vi "chart add series lv.vi"(7 "y2_axis":u8, 8 "error in (no error)":errorcluster, 9 "values":string, 10 "categories":string, 11 "chart":u32) -> (0 "error out":errorcluster, 3 "function return":u32)   [LabVIEW 8.6]
doc: "lxw_chart_series chart_add_series_lv(lxw_chart chart, const char *categories, const char *values, uint8_t y2_axis);"
uses:
  pending_lvxlsxwriter/xlsxwriter.dll
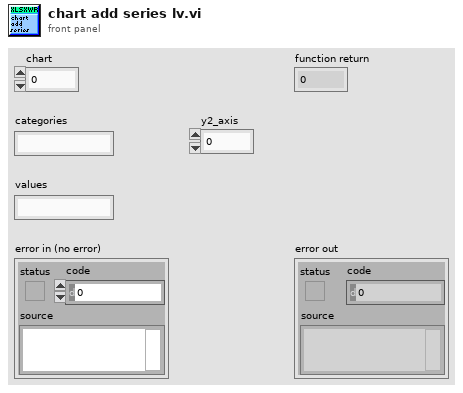
[diagram p1: front panel]
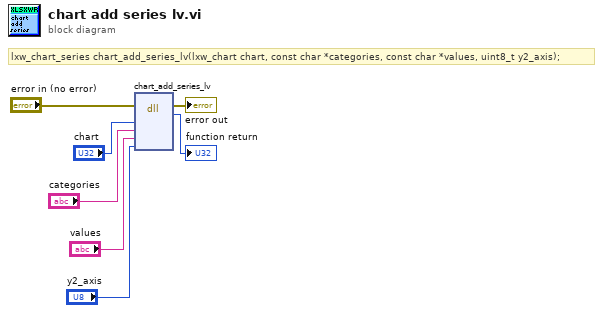
[diagram p0: block diagram]
diagram:
  # "lxw_chart_series chart_add_series_lv(lxw_chart chart, const char *categories, const char *values, uint8_t y2_axis);"
  n1 = dll-call lib="C:/Users/WDAGUtilityAccount/Desktop/pending_lvxlsxwriter/xlsxwriter.*" fn="chart_add_series_lv"(error in="error in (no error)", "chart"="chart", "categories"="categories", "values"="values", "y2_axis"="y2_axis") -> (error out=→"error out":errorcluster, →"function return":u32)  [unwired: 6 in, 1 out]
